vi "Generate PRBS AXIS Data.vi"(6 "ready for output":bool, 7 "reset":bool, 10 "enable":bool, 11 "number of lanes":u8) -> (0 "tlast":bool, 1 "tvalid":bool, 2 "tkeep":bool[](array[boolean]), 3 "tdata":bool[](array[boolean]))   [LabVIEW 2023, in "Aurora64b66b Utilities FPGA.lvlib"]
uses:
  Aurora64b66b Utilities FPGA.lvlib
  Program Files/NI/LVAddons/niidl/1/instr.lib/_niInstr/Data Formatting/v1/FPGA/niInstr Data Formatting v1 FPGA.lvlib
  Program Files/NI/LVAddons/niidl/1/instr.lib/_niInstr/Data Formatting/v1/FPGA/Private/Convert/U64 array to Boolean Array.vi
  Program Files/NI/LVAddons/niidl/1/instr.lib/_niInstr/Basic Elements/v1/FPGA/niInstr Basic Elements v1 FPGA.lvlib
  SubVIs/PRBS64 Parallel Tx - 8 Lanes.vi
  SubVIs/PRBS64 Parallel Tx - 4 Lanes.vi
  SubVIs/PRBS64 Parallel Tx - 16 Lanes.vi
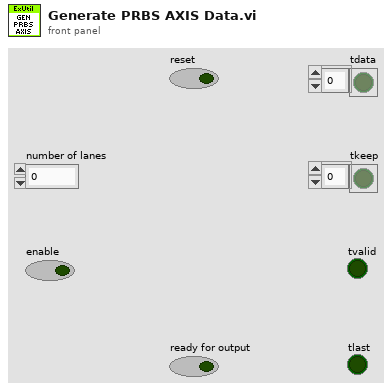
[diagram p1: front panel]
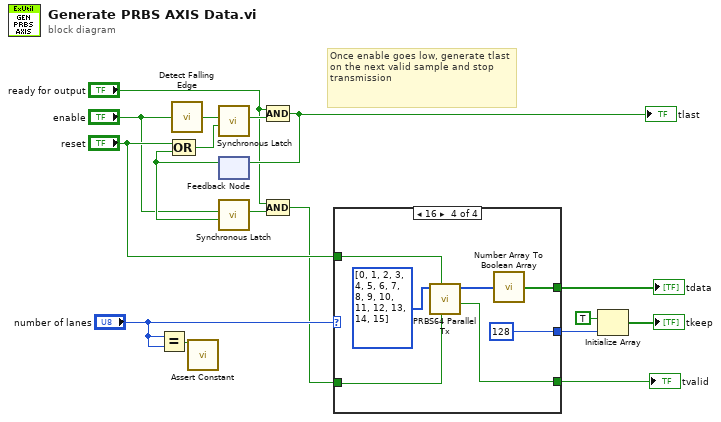
[diagram p0: block diagram]
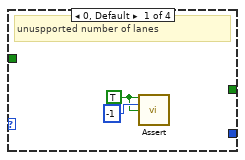
[diagram p2: hidden frame]
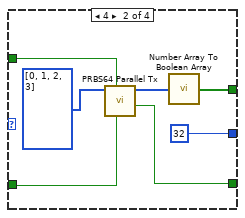
[diagram p3: hidden frame]
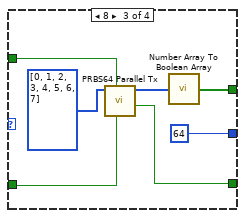
[diagram p4: hidden frame]
diagram:
  # "Once enable goes low, generate tlast on the next valid sample and stop transmission"
  n1 = Equal?(x="number of lanes", y="number of lanes") -> (x = y?=w13:bool)
  n2 = call "Detect Falling Edge.vi"("signal"="enable") -> ("edge detected"=w7:bool)  [unwired: 14 in]
  n3 = call "Assert Constant.vi"("constant terminal"=w13) -> ()  [unwired: 15 in]
  n4 = feedback #1() -> (w5:bool)  [unwired: 1 in]
  n5 = Compound Arithmetic op=OR("reset", w5) -> (w8:bool)
  n6 = call "Synchronous Latch.vi"("clear"=w8, "set"=w7) -> ("out"=w10:bool)  [unwired: 9 in]
  n7 = call "Synchronous Latch.vi"("clear"=w5, "set"="enable") -> ("out"=w4:bool)  [unwired: 9 in]
  n8 = Compound Arithmetic op=AND("ready for output", w10) -> (w9:bool)
  "tlast" <- w9
  n9 = feedback-in #1(w9) -> ()
  n10 = Compound Arithmetic op=AND("ready for output", w4) -> (w2:bool)
  n11 = case shown="16" "number of lanes" {
    tunnel: w2 -> [_ w21 w27 w34]
    tunnel: [_ w22 w28 w35] -> w16
    tunnel: [_ w23 w29 w36] -> w12
    tunnel: "reset" -> [_ w25 w31 w38]
    tunnel: [_ 32 ("dimension size") 64 ("dimension size") 128 ("dimension size")] -> w11
    frame 0, Default {
      w18 = TRUE ("assert")
      # "unuspported number of lanes"
      n12 = call "Assert.vi"("assert"=w18, "error code"=-1, "enable show error"=w18) -> ()  [unwired: 13 in]
    }
    frame 4 {
      n13 = call-poly "PRBS64 Parallel Tx.vi"("ready for output (T)"=w21, "reset"=w25, "seed"=u64[] [0, 1, 2, 3]) -> ("output valid"=w23:bool, "sequence out"=w24:u64[])  [unwired: 7 in]
      n14 = call-poly "Number Array To Boolean Array.vi"("data in"=w24) -> ("data out"=w22:bool[])  [unwired: 14 in]
    }
    frame 8 {
      n15 = call-poly "PRBS64 Parallel Tx.vi"("ready for output (T)"=w27, "reset"=w31, "seed"=u64[] [0, 1, 2, 3, 4, 5, 6, 7]) -> ("output valid"=w29:bool, "sequence out"=w30:u64[])  [unwired: 7 in]
      n16 = call-poly "Number Array To Boolean Array.vi"("data in"=w30) -> ("data out"=w28:bool[])  [unwired: 14 in]
    }
    frame 16 {
      n17 = call-poly "PRBS64 Parallel Tx.vi"("ready for output (T)"=w34, "reset"=w38, "seed"=u64[] [0, 1, 2, 3, 4, 5, 6, 7, 8, 9, 10, 11, 12, 13, 14, 15]) -> ("output valid"=w36:bool, "sequence out"=w37:u64[])  [unwired: 7 in]
      n18 = call-poly "Number Array To Boolean Array.vi"("data in"=w37) -> ("data out"=w35:bool[])  [unwired: 14 in]
    }
  }
  "tdata" <- w16
  "tvalid" <- w12
  n19 = Initialize Array(TRUE, w11) -> (→"tkeep":bool[])
